vi "Configure Bus Source (I2C).vi"(0 "VISA resource name":refnum<visa-resource-name>, 5 "BUS Number (9: Bus 1)":u16(ring)=9 items=["Bus 1"=9, "Bus 2"=10, "Bus 3"=11, "Bus 4"=12], 7 "Clock Source (0: Channel 1)":u16(ring) items=["Channel 1"=0, "Channel 2"=1, "Channel 3"=2, "Channel 4"=3, "Digital Channel 0"=14, "Digital Channel 1"=15, "Digital Channel 2"=16, "Digital Channel 3"=17, "Digital Channel 4"=18, "Digital Channel 5"=19, "Digital Channel 6"=20, "Digital Channel 7"=21, "Digital Channel 8"=22, "Digital Channel 9"=23, "Digital Channel 10"=24, "Digital Channel 11"=25, "Digital Channel 12"=26, "Digital Channel 13"=27, "Digital Channel 14"=28, "Digital Channel 15"=29], 9 "Data Source (1: Channel 2)":u16(ring)=1 items=["Channel 1"=0, "Channel 2"=1, "Channel 3"=2, "Channel 4"=3, "Digital Channel 0"=14, "Digital Channel 1"=15, "Digital Channel 2"=16, "Digital Channel 3"=17, "Digital Channel 4"=18, "Digital Channel 5"=19, "Digital Channel 6"=20, "Digital Channel 7"=21, "Digital Channel 8"=22, "Digital Channel 9"=23, "Digital Channel 10"=24, "Digital Channel 11"=25, "Digital Channel 12"=26, "Digital Channel 13"=27, "Digital Channel 14"=28, "Digital Channel 15"=29], 11 "error in (no error)":errorcluster, 12 "Enable R/W Inclusion In Address (F: Disable)":bool) -> (4 "VISA resource name out":refnum<visa-resource-name>, 15 "error out":errorcluster)   [LabVIEW 2016, in "Tektronix DPO MSO 2000 4000 Series.lvlib"]
doc: "Configures I2C bus settings for an oscilloscope.\n\n<B>Note:</B>\nThe <B>MDO4000C series</B>, only has a maximum of <B>3</B> busses, whereas older 4000 series had up to <B>4</B>."
uses:
  Tektronix DPO MSO 2000 4000 Series.lvlib
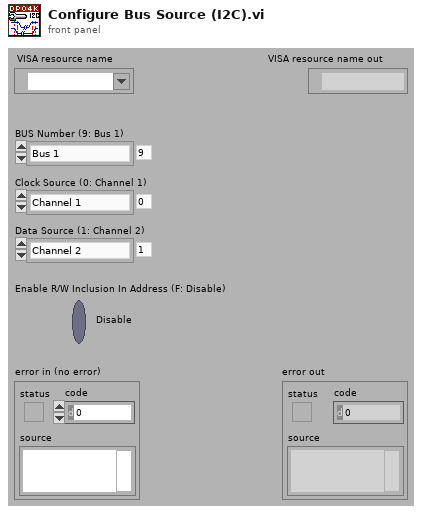
[diagram p1: front panel]
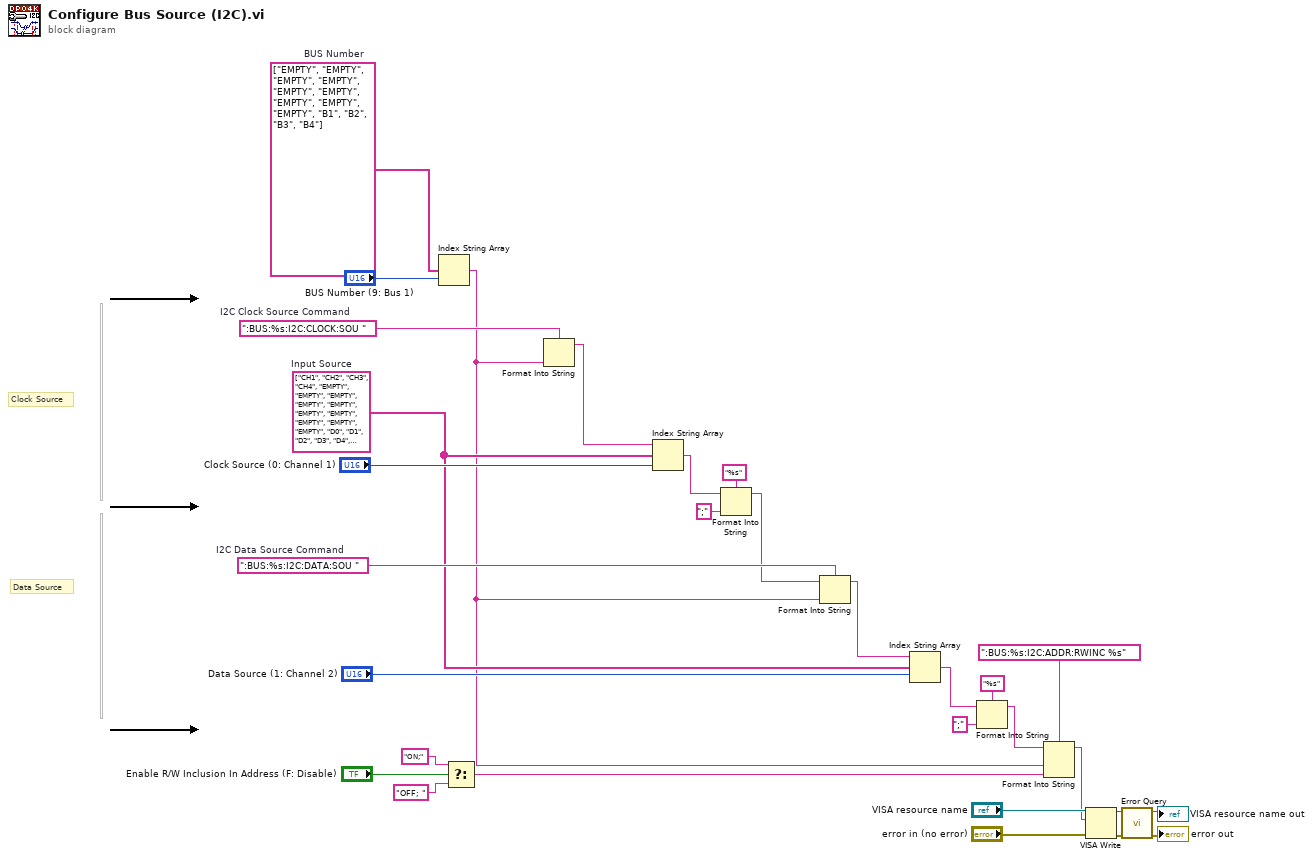
[diagram p0: block diagram]
diagram:
  w9 = string[] ["CH1", "CH2", "CH3", "CH4", "EMPTY", "EMPTY", "EMPTY", "EMPTY", "EMPTY", "EMPTY", "EMPTY", "EMPTY", "EMPTY", "EMPTY", "D0", "D1", "D2", "D3", "D4", "D5", "D6", "D7", "D8", "D9", "D10", "D11", "D12", "D13", "D14", "D15"]  # Input Source
  w27 = ":BUS:%s:I2C:DATA:SOU "  # I2C Data Source Command
  w29 = ":BUS:%s:I2C:CLOCK:SOU "  # I2C Clock Source Command
  w20 = string[] ["EMPTY", "EMPTY", "EMPTY", "EMPTY", "EMPTY", "EMPTY", "EMPTY", "EMPTY", "EMPTY", "B1", "B2", "B3", "B4"]  # BUS Number
  # "Data Source"
  # "Clock Source"
  n1 = Index String Array(1:"BUS Number (9: Bus 1)", 2:w20) -> (0:w5:string)  [unwired: 1 in]
  n2 = Select(t="ON;" ("format string"), s="Enable R/W Inclusion In Address (F: Disable)", f="OFF; " ("format string")) -> (s? t:f=w6:string)
  n3 = Format Into String(format string=w29, w5) -> (resulting string=w25:string)  [unwired: 2 in, 1 out]
  n4 = Index String Array(1:"Clock Source (0: Channel 1)", 2:w9, 3:w25) -> (0:w15:string)
  n5 = Format Into String(format string="%s", initial string=w15, ";" ("input 1")) -> (resulting string=w23:string)  [unwired: 1 in, 1 out]
  n6 = Format Into String(format string=w27, initial string=w23, w5) -> (resulting string=w22:string)  [unwired: 1 in, 1 out]
  n7 = Index String Array(1:"Data Source (1: Channel 2)", 2:w9, 3:w22) -> (0:w13:string)
  n8 = Format Into String(format string="%s", initial string=w13, ";" ("input 1")) -> (resulting string=w8:string)  [unwired: 1 in, 1 out]
  n9 = Format Into String(format string=":BUS:%s:I2C:ADDR:RWINC %s", initial string=w8, w5, w6) -> (resulting string=w1:string)  [unwired: 1 in, 1 out]
  n10 = VISA Write(VISA resource name="VISA resource name", write buffer=w1, error in (no error)="error in (no error)") -> (VISA resource name out=w19:refnum<visa-resource-name>, error out=w18:errorcluster)  [unwired: 1 out]
  n11 = call "Error Query.vi"("error in (no error)"=w18, "VISA resource name"=w19) -> ("error out"=→"error out":errorcluster, "VISA resource name out"=→"VISA resource name out":refnum<visa-resource-name>)  [unwired: 6 in, 2 out]
